vi "Approximately equal - percent of target.vi"(9 "% tolerance":dbl=1.0 format="%.2f", 10 "actual":dbl=99.0 format="%.5e", 11 "target":dbl=100.0 format="%.5e") -> (1 "delta":dbl=1.0, 2 "equal?":bool=TRUE)   [LabVIEW 2013]
doc: "Is target and actual equal within % tolerance?"
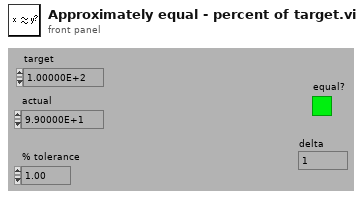
[diagram p1: front panel]
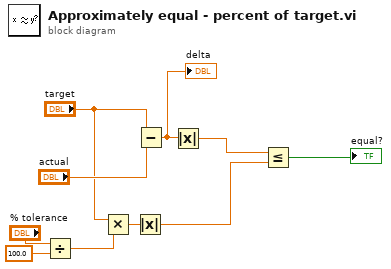
[diagram p0: block diagram]
diagram:
  n1 = Divide(x="% tolerance", y=100.0) -> (x/y=w4:dbl)
  n2 = Multiply(x="target", y=w4) -> (x*y=w2:dbl)
  n3 = Absolute Value(x=w2) -> (abs(x)=w1:dbl)
  n4 = Subtract(x="target", y="actual") -> (x-y=w8:dbl)
  "delta" <- w8
  n5 = Absolute Value(x=w8) -> (abs(x)=w10:dbl)
  n6 = Less Or Equal?(x=w10, y=w1) -> (x <= y?=→"equal?":bool)
